vi "定点周期设置.vi"(6 "启用参数":T1={"氨氮"=TRUE, "总磷"=TRUE, "总氮"=TRUE, "CODMn"=TRUE, "CODCr"=TRUE} caption="测量参数", 8 "测量参数":T1={"氨氮"=TRUE, "总磷"=TRUE, "总氮"=TRUE, "CODMn"=TRUE, "CODCr"=TRUE}, 9 "间隔启动":T6 {"启动命令" items=["", "加标回收（启动采配水）", "加标回收（不启动采配水）", "水样测试（启动采配水）", "水样测试（不启动采配水）"]}, 10 "定点周期":T3 {"启动命令 24" items=["", "加标回收（启动采配水）", "加标回收（不启动采配水）", "水样测试（启动采配水）", "水样测试（不启动采配水）"]; "启动命令 23" items=["", "加标回收（启动采配水）", "加标回收（不启动采配水）", "水样测试（启动采配水）", "水样测试（不启动采配水）"]; "启动命令 22" items=["", "加标回收（启动采配水）", "加标回收（不启动采配水）", "水样测试（启动采配水）", "水样测试（不启动采配水）"]; "启动命令 21" items=["", "加标回收（启动采配水）", "加标回收（不启动采配水）", "水样测试（启动采配水）", "水样测试（不启动采配水）"]; "启动命令 20" items=["", "加标回收（启动采配水）", "加标回收（不启动采配水）", "水样测试（启动采配水）", "水样测试（不启动采配水）"]; "启动命令 19" items=["", "加标回收（启动采配水）", "加标回收（不启动采配水）", "水样测试（启动采配水）", "水样测试（不启动采配水）"]; "启动命令 18" items=["", "加标回收（启动采配水）", "加标回收（不启动采配水）", "水样测试（启动采配水）", "水样测试（不启动采配水）"]; "启动命令 17" items=["", "加标回收（启动采配水）", "加标回收（不启动采配水）", "水样测试（启动采配水）", "水样测试（不启动采配水）"]; "启动命令 16" items=["", "加标回收（启动采配水）", "加标回收（不启动采配水）", "水样测试（启动采配水）", "水样测试（不启动采配水）"]; "启动命令 15" items=["", "加标回收（启动采配水）", "加标回收（不启动采配水）", "水样测试（启动采配水）", "水样测试（不启动采配水）"]; "启动命令 14" items=["", "加标回收（启动采配水）", "加标回收（不启动采配水）", "水样测试（启动采配水）", "水样测试（不启动采配水）"]; "启动命令 13" items=["", "加标回收（启动采配水）", "加标回收（不启动采配水）", "水样测试（启动采配水）", "水样测试（不启动采配水）"]; "启动命令 12" items=["", "加标回收（启动采配水）", "加标回收（不启动采配水）", "水样测试（启动采配水）", "水样测试（不启动采配水）"]; "启动命令 11" items=["", "加标回收（启动采配水）", "加标回收（不启动采配水）", "水样测试（启动采配水）", "水样测试（不启动采配水）"]; "启动命令 10" items=["", "加标回收（启动采配水）", "加标回收（不启动采配水）", "水样测试（启动采配水）", "水样测试（不启动采配水）"]; "启动命令 9" items=["", "加标回收（启动采配水）", "加标回收（不启动采配水）", "水样测试（启动采配水）", "水样测试（不启动采配水）"]; "启动命令 8" items=["", "加标回收（启动采配水）", "加标回收（不启动采配水）", "水样测试（启动采配水）", "水样测试（不启动采配水）"]; "启动命令 7" items=["", "加标回收（启动采配水）", "加标回收（不启动采配水）", "水样测试（启动采配水）", "水样测试（不启动采配水）"]; "启动命令 6" items=["", "加标回收（启动采配水）", "加标回收（不启动采配水）", "水样测试（启动采配水）", "水样测试（不启动采配水）"]; "启动命令 5" items=["", "加标回收（启动采配水）", "加标回收（不启动采配水）", "水样测试（启动采配水）", "水样测试（不启动采配水）"]; "启动命令 4" items=["", "加标回收（启动采配水）", "加标回收（不启动采配水）", "水样测试（启动采配水）", "水样测试（不启动采配水）"]; "启动命令 3" items=["", "加标回收（启动采配水）", "加标回收（不启动采配水）", "水样测试（启动采配水）", "水样测试（不启动采配水）"]; "启动命令 2" items=["", "加标回收（启动采配水）", "加标回收（不启动采配水）", "水样测试（启动采配水）", "水样测试（不启动采配水）"]; "启动命令" items=["", "加标回收（启动采配水）", "加标回收（不启动采配水）", "水样测试（启动采配水）", "水样测试（不启动采配水）"]}, 11 "周期模式":T2) -> (2 "保存输出":bool, 3 "周期设置输出":T5={"周期模式"=enum."不启用", "定点周期"={"启动命令"=0, "启动命令 2"=0, "启动命令 3"=0, "启动命令 4"=0, "启动命令 5"=0, "启动命令 6"=0, "启动命令 7"=0, "启动命令 8"=0, "启动命令 9"=0, "启动命令 10"=0, "启动命令 11"=0, "启动命令 12"=0, "启动命令 13"=0, "启动命令 14"=0, "启动命令 15"=0, "启动命令 16"=0, "启动命令 17"=0, "启动命令 18"=0, "启动命令 19"=0, "启动命令 20"=0, "启动命令 21"=0, "启动命令 22"=0, "启动命令 23"=0, "启动命令 24"=0}, "间隔设置"={"启动命令"=0, "启动间隔"=0.0, "启动次数"=0}, "测量参数"={"氨氮"=TRUE, "总磷"=TRUE, "总氮"=TRUE, "CODMn"=TRUE, "CODCr"=TRUE}} {"定点周期"."启动命令 24" items=["", "加标回收（启动采配水）", "加标回收（不启动采配水）", "水样测试（启动采配水）", "水样测试（不启动采配水）"]; "定点周期"."启动命令 23" items=["", "加标回收（启动采配水）", "加标回收（不启动采配水）", "水样测试（启动采配水）", "水样测试（不启动采配水）"]; "定点周期"."启动命令 22" items=["", "加标回收（启动采配水）", "加标回收（不启动采配水）", "水样测试（启动采配水）", "水样测试（不启动采配水）"]; "定点周期"."启动命令 21" items=["", "加标回收（启动采配水）", "加标回收（不启动采配水）", "水样测试（启动采配水）", "水样测试（不启动采配水）"]; "定点周期"."启动命令 20" items=["", "加标回收（启动采配水）", "加标回收（不启动采配水）", "水样测试（启动采配水）", "水样测试（不启动采配水）"]; "定点周期"."启动命令 19" items=["", "加标回收（启动采配水）", "加标回收（不启动采配水）", "水样测试（启动采配水）", "水样测试（不启动采配水）"]; "定点周期"."启动命令 18" items=["", "加标回收（启动采配水）", "加标回收（不启动采配水）", "水样测试（启动采配水）", "水样测试（不启动采配水）"]; "定点周期"."启动命令 17" items=["", "加标回收（启动采配水）", "加标回收（不启动采配水）", "水样测试（启动采配水）", "水样测试（不启动采配水）"]; "定点周期"."启动命令 16" items=["", "加标回收（启动采配水）", "加标回收（不启动采配水）", "水样测试（启动采配水）", "水样测试（不启动采配水）"]; "定点周期"."启动命令 15" items=["", "加标回收（启动采配水）", "加标回收（不启动采配水）", "水样测试（启动采配水）", "水样测试（不启动采配水）"]; "定点周期"."启动命令 14" items=["", "加标回收（启动采配水）", "加标回收（不启动采配水）", "水样测试（启动采配水）", "水样测试（不启动采配水）"]; "定点周期"."启动命令 13" items=["", "加标回收（启动采配水）", "加标回收（不启动采配水）", "水样测试（启动采配水）", "水样测试（不启动采配水）"]; "定点周期"."启动命令 12" items=["", "加标回收（启动采配水）", "加标回收（不启动采配水）", "水样测试（启动采配水）", "水样测试（不启动采配水）"]; "定点周期"."启动命令 11" items=["", "加标回收（启动采配水）", "加标回收（不启动采配水）", "水样测试（启动采配水）", "水样测试（不启动采配水）"]; "定点周期"."启动命令 10" items=["", "加标回收（启动采配水）", "加标回收（不启动采配水）", "水样测试（启动采配水）", "水样测试（不启动采配水）"]; "定点周期"."启动命令 9" items=["", "加标回收（启动采配水）", "加标回收（不启动采配水）", "水样测试（启动采配水）", "水样测试（不启动采配水）"]; "定点周期"."启动命令 8" items=["", "加标回收（启动采配水）", "加标回收（不启动采配水）", "水样测试（启动采配水）", "水样测试（不启动采配水）"]; "定点周期"."启动命令 7" items=["", "加标回收（启动采配水）", "加标回收（不启动采配水）", "水样测试（启动采配水）", "水样测试（不启动采配水）"]; "定点周期"."启动命令 6" items=["", "加标回收（启动采配水）", "加标回收（不启动采配水）", "水样测试（启动采配水）", "水样测试（不启动采配水）"]; "定点周期"."启动命令 5" items=["", "加标回收（启动采配水）", "加标回收（不启动采配水）", "水样测试（启动采配水）", "水样测试（不启动采配水）"]; "定点周期"."启动命令 4" items=["", "加标回收（启动采配水）", "加标回收（不启动采配水）", "水样测试（启动采配水）", "水样测试（不启动采配水）"]; "定点周期"."启动命令 3" items=["", "加标回收（启动采配水）", "加标回收（不启动采配水）", "水样测试（启动采配水）", "水样测试（不启动采配水）"]; "定点周期"."启动命令 2" items=["", "加标回收（启动采配水）", "加标回收（不启动采配水）", "水样测试（启动采配水）", "水样测试（不启动采配水）"]; "定点周期"."启动命令" items=["", "加标回收（启动采配水）", "加标回收（不启动采配水）", "水样测试（启动采配水）", "水样测试（不启动采配水）"]; "间隔设置"."启动命令" items=["", "加标回收（启动采配水）", "加标回收（不启动采配水）", "水样测试（启动采配水）", "水样测试（不启动采配水）"]})   [LabVIEW 2016, in "ZK定时设置.xctl"]
panel:
  in  "保存":bool
  in  "退出":bool
  in  "批量设置":bool
  out "周期模式选择卡":enum32{"选项卡 1", "选项卡 2"}(tab)
  # "分钟"
  # "次"
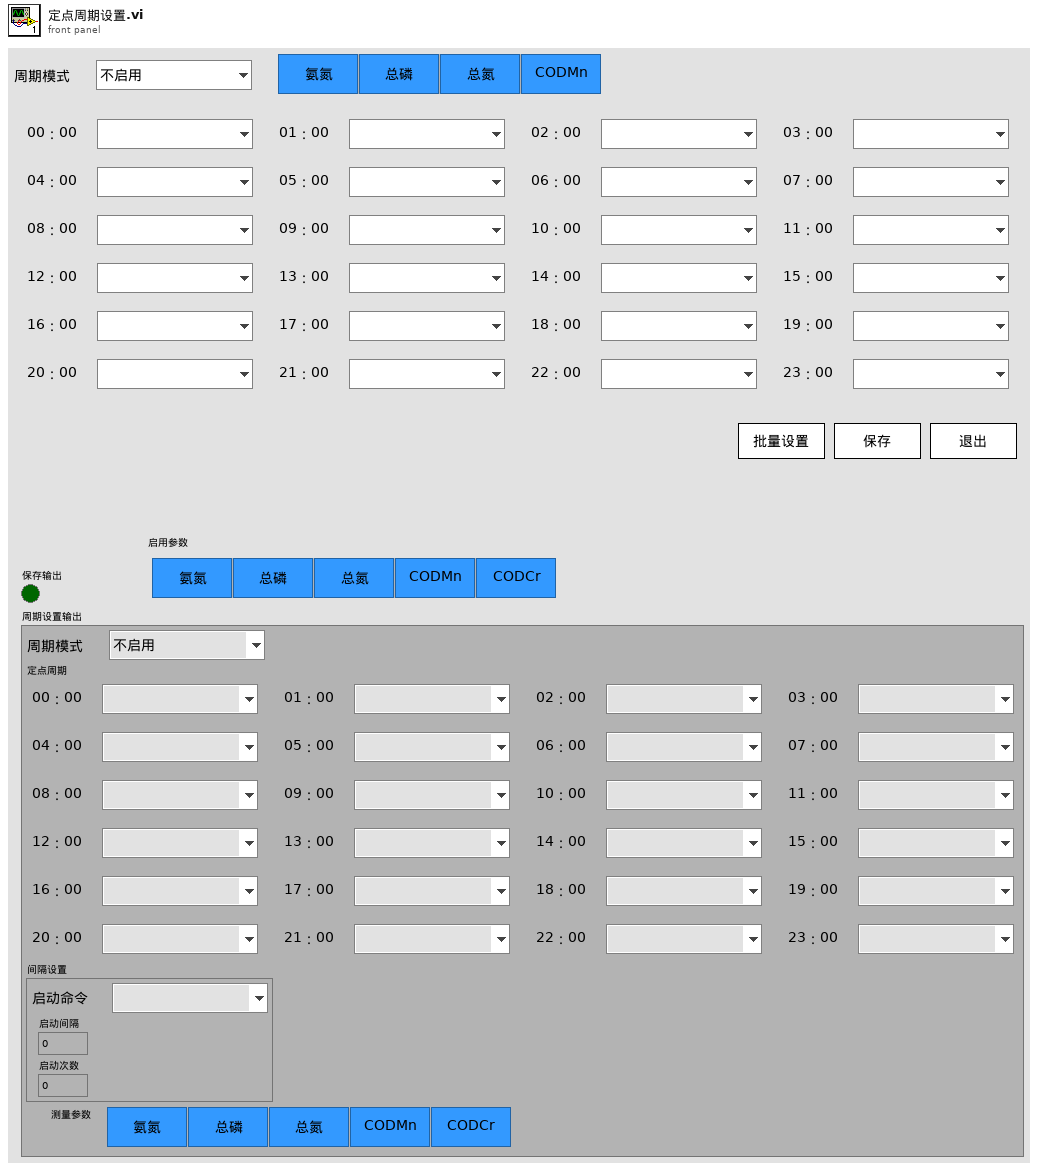
[diagram p1: front panel]
types:
  T1 = typedef "ZK定时设置.xctl/测量参数.ctl" = cluster{"氨氮":bool, "总磷":bool, "总氮":bool, "CODMn":bool, "CODCr":bool}
  T2 = typedef "ZK定时设置.xctl/周期模式设置.ctl" = enum16{"不启用", "定点模式", "间隔模式"}
  T3 = typedef "ZK定时设置.xctl/定点周期设置.ctl" = cluster{"启动命令":T4, "启动命令 2":T4, "启动命令 3":T4, "启动命令 4":T4, "启动命令 5":T4, "启动命令 6":T4, "启动命令 7":T4, "启动命令 8":T4, "启动命令 9":T4, "启动命令 10":T4, "启动命令 11":T4, "启动命令 12":T4, "启动命令 13":T4, "启动命令 14":T4, "启动命令 15":T4, "启动命令 16":T4, "启动命令 17":T4, "启动命令 18":T4, "启动命令 19":T4, "启动命令 20":T4, "启动命令 21":T4, "启动命令 22":T4, "启动命令 23":T4, "启动命令 24":T4}
  T4 = typedef "ZK定时设置.xctl/启动命令选择.ctl" = u16
  T5 = cluster{"周期模式":T2, "定点周期":T3, "间隔设置":cluster{"启动命令":T4, "启动间隔":dbl, "启动次数":i32}, "测量参数":T1}
  T6 = typedef "ZK定时设置.xctl/间隔启动设置.ctl" = cluster{"启动命令":T4, "启动间隔":dbl, "启动次数":i32}
  T7 = typedef "周期设置.lvlib/周期模式设置.ctl" = enum16{"不启用", "定点模式", "间隔模式"}
  T8 = cluster{"周期模式":T2, "定点周期":T3, cluster{"启动命令":T4, "启动间隔":dbl, "启动次数":i32}, "测量参数":T1}
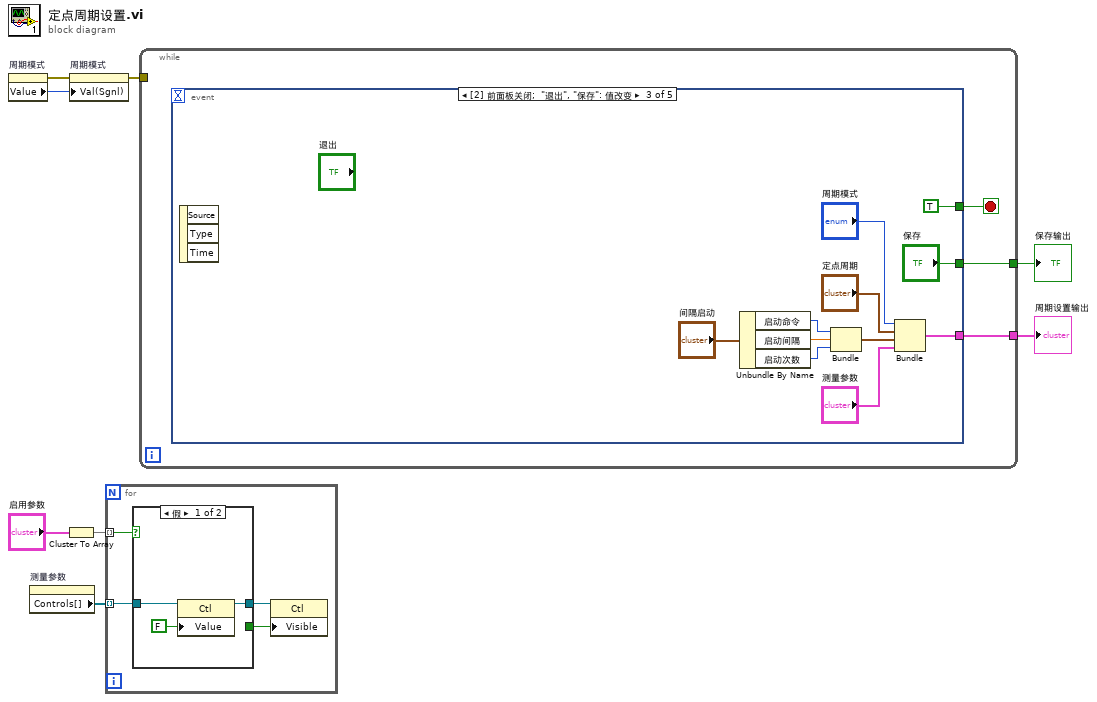
[diagram p0: block diagram]
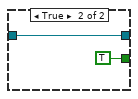
[diagram p2: hidden frame]
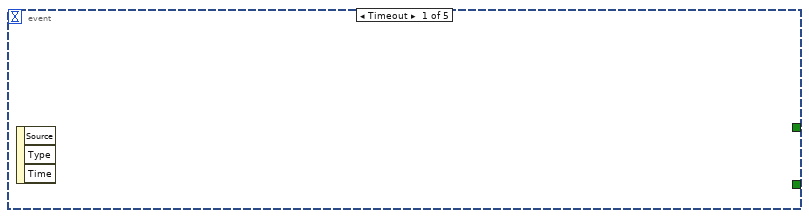
[diagram p3: hidden frame]
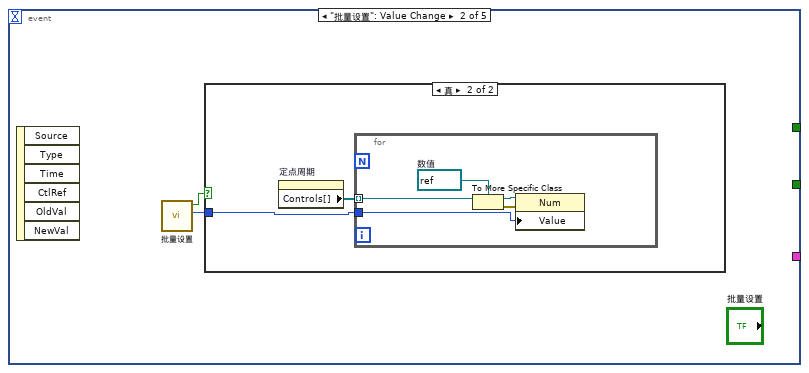
[diagram p4: hidden frame]
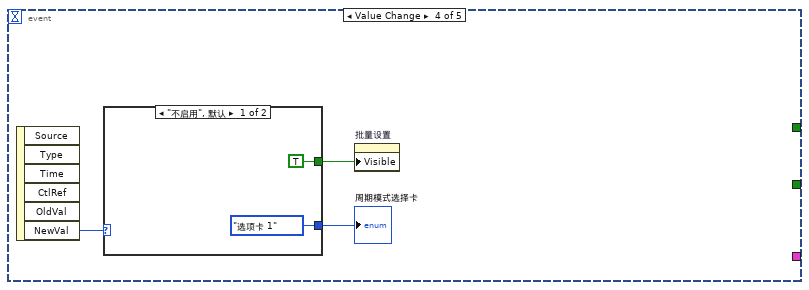
[diagram p6: hidden frame]
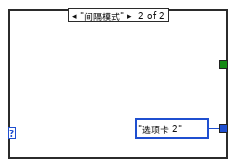
[diagram p7: hidden frame]
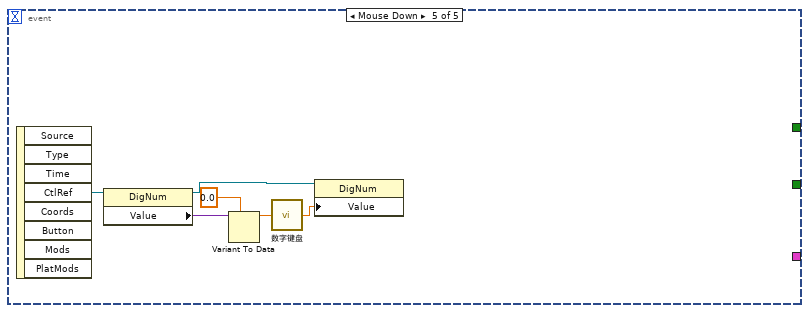
[diagram p8: hidden frame]
diagram:
  n1 = property on="周期模式" class="Enum (严格)"() -> (error out=w7:errorcluster, "Value"=w8:T7)  [unwired: 2 in, 1 out]
  n2 = property on="测量参数" class="Clust (严格)"() -> ("Controls[]"=w3:refnum<vi>[])  [unwired: 2 in, 2 out]
  n3 = Cluster To Array(cluster="启用参数") -> (array=w1:bool[])
  n4 = property on="周期模式" class="Enum (严格)"(error in=w7, "Val(Sgnl)"=w8) -> (error out=w6:errorcluster)  [unwired: 1 in, 1 out]
  n5 = for {
    tunnel: w3 -> [w10] mode=indexing
    tunnel: w1 -> [w12] mode=indexing
    n6 = case shown="假" w12 {
      tunnel: [w14 w17] -> w11
      tunnel: w10 -> [w15 w17]
      tunnel: [_ TRUE ("可见")] -> w9
      frame False {
        n7 = property class="Ctl"(reference=w15, "Value"=FALSE) -> (reference out=w14:refnum<vi>)  [unwired: 1 in, 1 out]
      }
      frame True {
      }
    }
    n8 = property class="Ctl"(reference=w11, "Visible"=w9) -> ()  [unwired: 1 in, 2 out]
  }
  n9 = while {
    tunnel: [w19] -> w5
    tunnel: w6 -> [_]
    tunnel: [w18] -> w4
    stop <- w20 stop-if-true
    n10 = event shown="[2] 前面板关闭;  \"退出\", \"保存\": 值改变" {
      selector: _ -> [_ _ _ _ _]
      dyn-events: _ -> [_ _ _ _ _]
      timeout: _ -> [_ _ _ _ _]
      tunnel: [_ _ TRUE _ _] -> w20
      tunnel: [_ _ w39 _ _] -> w19
      tunnel: [_ _ "保存" _ _] -> w18
      event Timeout {
        n11 = event-data() -> ()  [unwired: 1 in, 3 out]
      }
      event "批量设置": Value Change {
        n12 = event-data() -> ()  [unwired: 1 in, 6 out]
        n13 = call "批量设置.vi"() -> ("启动命令 2"=w22:T4, "确定 2"=w21:bool)  [unwired: 10 in]
        n14 = case shown="真" w21 {
          tunnel: w22 -> [_ w23]
          frame False {
          }
          frame True {
            n15 = property on="定点周期" class="Clust (严格)"() -> ("Controls[]"=w24:refnum<vi>[])  [unwired: 2 in, 2 out]
            n16 = for {
              tunnel: w24 -> [w29] mode=indexing
              tunnel: w23 -> [w25]
              w28 = refnum<vi> refnum  # 数值
              n17 = To More Specific Class(target class=w28, reference=w29) -> (specific class reference=w27:refnum<vi>, error out=w26:errorcluster)  [unwired: 1 in]
              n18 = property class="Num"(reference=w27, error in=w26, "Value"=w25) -> ()  [unwired: 2 out]
            }
          }
        }
      }
      event Panel Close; "退出", "保存": Value Change {
        n19 = event-data() -> ()  [unwired: 1 in, 3 out]
        n20 = Unbundle By Name("间隔启动") -> ("启动命令"=w36:T4, "启动间隔"=w35:dbl, "启动次数"=w34:i32)
        n21 = Bundle("启动命令"=w36, "启动间隔"=w35, "启动次数"=w34) -> (w33:cluster{"启动命令":T4, "启动间隔":dbl, "启动次数":i32})  [unwired: 1 in]
        n22 = Bundle("周期模式"="周期模式", "定点周期"="定点周期", w33, "测量参数"="测量参数") -> (w39:T8)  [unwired: 1 in]
      }
      event Value Change {
        n23 = event-data() -> ("NewVal"=w42:T2)  [unwired: 1 in, 5 out]
        n24 = case shown="\"不启用\", 默认" w42 {
          tunnel: [TRUE ("可见") _] -> w43
          tunnel: [enum32{"选项卡 1", "选项卡 2"}."选项卡 1" ("周期模式选择卡") enum32{"选项卡 1", "选项卡 2"}."选项卡 2" ("周期模式选择卡")] -> w41
          frame "不启用", Default {
          }
          frame "间隔模式" {
          }
        }
        "周期模式选择卡" <- w41
        n25 = property on="批量设置" class="Bool"("Visible"=w43) -> ()  [unwired: 2 in, 2 out]
      }
      event Mouse Down {
        n26 = event-data() -> ("CtlRef"=w52:refnum<vi>)  [unwired: 1 in, 7 out]
        n27 = property class="DigNum"(reference=w52) -> (reference out=w51:refnum<vi>, "Value"=w50:variant)  [unwired: 1 in, 1 out]
        n28 = Variant To Data(type=0.0, Variant=w50) -> (data=w48:dbl)  [unwired: 1 in, 1 out]
        n29 = call "数字键盘.vi"("OldNumber"=w48) -> ("NewNumber"=w47:sgl)
        n30 = property class="DigNum"(reference=w51, "Value"=w47) -> ()  [unwired: 1 in, 2 out]
      }
    }
  }
  "周期设置输出" <- w5
  "保存输出" <- w4
